vi "SendACC.vi"(8 "error in (no error)":errorcluster, 10 "appended array":T1[](array[typedef]), 11 "Database ref":refnum<k24>) -> (0 "error out":errorcluster)   [LabVIEW 2015]
uses:
  C:/Users/Bartek/Desktop/NORDIC Labview GUI/DLLs/NordicDatabaseDLL.dll
  DLLs/NordicDatabaseDLL.dll
  ctrls/AccelerometerData.ctl
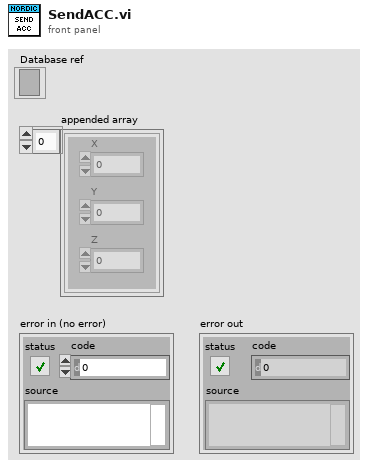
[diagram p1: front panel]
types:
  T1 = typedef "AccelerometerData.ctl" = cluster{"X":dbl, "Y":dbl, "Z":dbl}
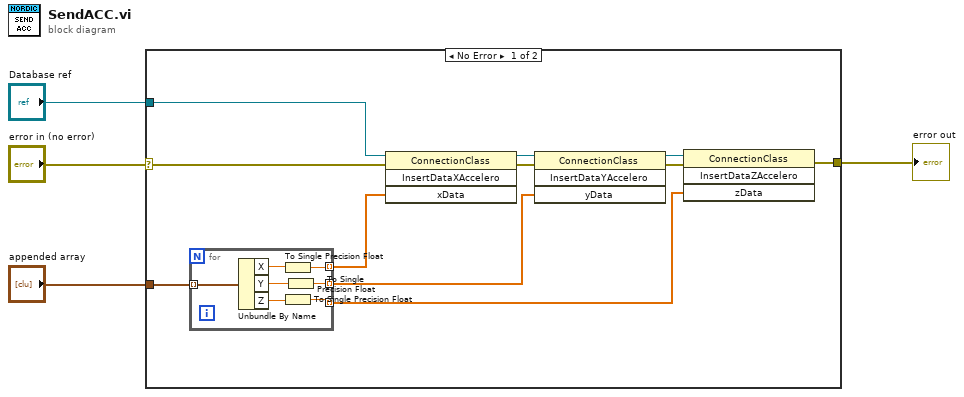
[diagram p0: block diagram]
diagram:
  n1 = case shown="No Error" "error in (no error)" {
    selector: "error in (no error)" -> [w14 w23]
    tunnel: [w5 w23] -> w3
    tunnel: "Database ref" -> [w15 _]
    tunnel: "appended array" -> [w13 _]
    frame No Error {
      n2 = for {
        tunnel: w13 -> [w22] mode=indexing
        tunnel: [w20] -> w12 mode=indexing
        tunnel: [w17] -> w9 mode=indexing
        tunnel: [w16] -> w6 mode=indexing
        n3 = Unbundle By Name(w22) -> ("X"=w21:dbl, "Y"=w19:dbl, "Z"=w18:dbl)
        n4 = To Single Precision Float(number=w21) -> (single precision float=w20:sgl)
        n5 = To Single Precision Float(number=w18) -> (single precision float=w16:sgl)
        n6 = To Single Precision Float(number=w19) -> (single precision float=w17:sgl)
      }
      n7 = invoke class="ConnectionClass" method="InsertDataXAccelero"(reference=w15, error in=w14, "xData"=w12) -> (reference out=w7:refnum<k24>, error out=w8:errorcluster)  [unwired: 1 in, 2 out]
      n8 = invoke class="ConnectionClass" method="InsertDataYAccelero"(reference=w7, error in=w8, "yData"=w9) -> (reference out=w11:refnum<k24>, error out=w10:errorcluster)  [unwired: 1 in, 2 out]
      n9 = invoke class="ConnectionClass" method="InsertDataZAccelero"(reference=w11, error in=w10, "zData"=w6) -> (error out=w5:errorcluster)  [unwired: 1 in, 3 out]
    }
    frame Error {
    }
  }
  "error out" <- w3
